vi "Quiz6.vi"() -> ()   [LabVIEW 2017]
panel:
  out "จำนวนรอบLED":i32
  out "?":bool
  out "นับรอบ":i32
  in  "Start":bool
  in  "stop":bool
  out "Numeric 2":dbl
  out "Boolean 3":bool
  in  "Stop 2":bool
  in  "Boolean 2":bool
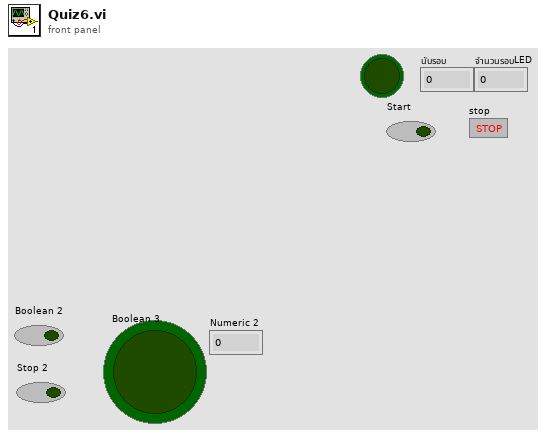
[diagram p1: front panel]
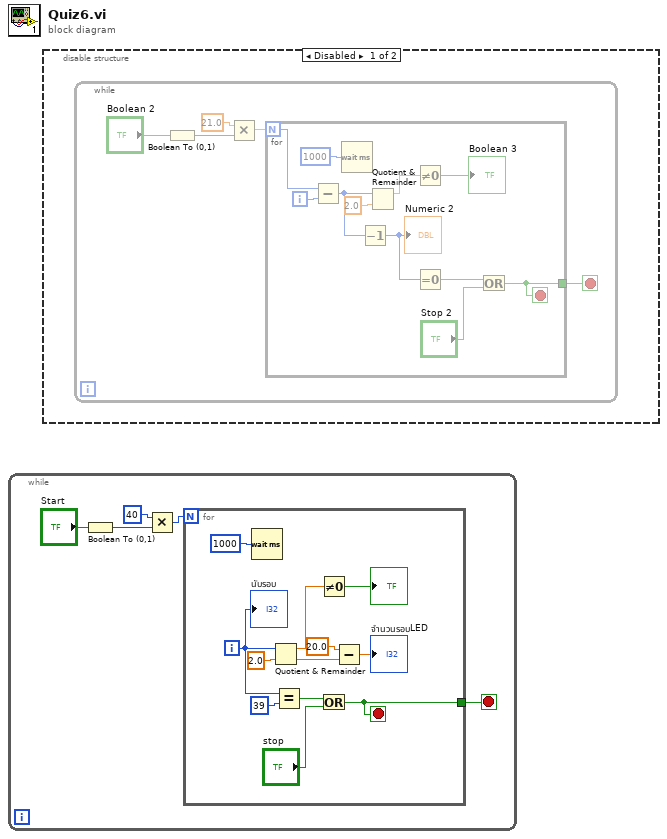
[diagram p0: block diagram]
diagram:
  n1 = while {
    stop <- w5 stop-if-true
    n2 = Boolean To (0,1)(Boolean="Start") -> (0, 1=w3:i16)
    n3 = Multiply(x=i16 40, y=w3) -> (x*y=w4:i16)
    n4 = for {
      N: w4 -> [_]
      tunnel: [w16] -> w5
      i -> [w10]
      stop <- w16 stop-if-true
      n5 = Wait (ms)(milliseconds to wait=u32 1000) -> ()  [unwired: 1 out]
      n6 = Quotient & Remainder(x=w10, y=2.0) -> (x-y*floor(x/y)=w14:dbl, floor(x/y)=w8:dbl)
      n7 = Equal?(x=w10, y=39) -> (x = y?=w12:bool)
      n8 = Not Equal To 0?(x=w14) -> (x != 0?=→"?":bool)
      n9 = Or(x=w12, y="stop") -> (x .or. y?=w16:bool)
      n10 = Subtract(x=20.0, y=w8) -> (x-y=→"จำนวนรอบLED":dbl)
      "นับรอบ" <- w10
    }
  }
  n11 = disable-structure shown="Disabled" {
    frame Disabled {
      n12 = while {
        stop <- w18 stop-if-true
        n13 = Boolean To (0,1)(Boolean="Boolean 2") -> (0, 1=w19:i16)
        n14 = Multiply(x=21.0 ("value"), y=w19) -> (x*y=w21:dbl)
        n15 = for {
          N: w21 -> [w25]
          tunnel: [w23] -> w18
          i -> [w26]
          stop <- w23 stop-if-true
          n16 = Subtract(x=w25, y=w26) -> (x-y=w31:i32)
          n17 = Wait (ms)(milliseconds to wait=u32 1000 ("millisecond timer value")) -> ()  [unwired: 1 out]
          n18 = Decrement(x=w31) -> (x-1=w24:i32)
          "Numeric 2" <- w24
          n19 = Quotient & Remainder(x=w31, y=2.0) -> (x-y*floor(x/y)=w29:dbl)  [unwired: 1 out]
          n20 = Not Equal To 0?(x=w29) -> (x != 0?=→"Boolean 3":bool)
          n21 = Equal To 0?(x=w24) -> (x = 0?=w32:bool)
          n22 = Or(x=w32, y="Stop 2") -> (x .or. y?=w23:bool)
        }
      }
    }
    frame Enabled {
    }
  }
